vi "GetCrossSpectrumPhase.vi"(6 "calc cache":variant, 8 "error in (no error)":errorcluster, 10 "speed profile (positions [s])":sgl[](array[numeric]), 11 "waveform":waveform(sgl)) -> (0 "error out":errorcluster, 2 "channel name":string, 3 "cross phase [degrees]":cluster{"f0":dbl, "df":dbl, "phase":sgl[]}, 4 "calc cache out":variant)   [LabVIEW 2017]
uses:
  <vilib>/addons/InsightCM/Utilities/Analysis/Vibration/VibrationAnalysisFunctions.lvlib
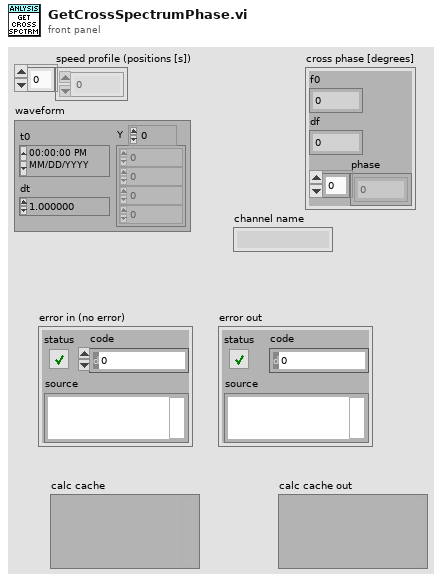
[diagram p1: front panel]
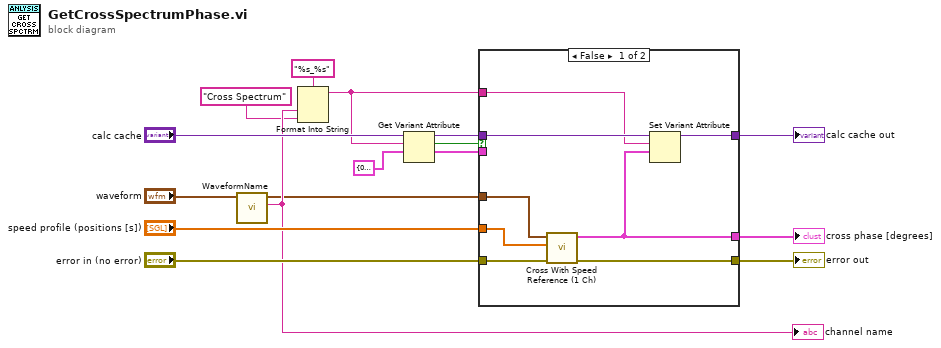
[diagram p0: block diagram]
diagram:
  n1 = call <vilib>:"WaveformName.vi"("signal in"="waveform") -> ("name"=w5:string, "signal out"=w3:waveform(sgl))  [unwired: 9 in]
  "channel name" <- w5
  n2 = Format Into String(format string="%s_%s", w5, "Cross Spectrum" ("name")) -> (resulting string=w1:string)  [unwired: 2 in, 1 out]
  n3 = Get Variant Attribute(Variant="calc cache", name=w1, default value (empty Variant)=cluster{"f0":dbl, "df":dbl, "phase":sgl[]} {"f0"=0.0, "df"=0.0, "phase"=[]} ("Cross phase [degrees]")) -> (duplicate Variant=w11:variant, found=w8:bool, value=w7:cluster{"f0":dbl, "df":dbl, "phase":sgl[]})  [unwired: 1 in, 1 out]
  n4 = case shown="False" w8 {
    tunnel: "error in (no error)" -> [w24 w27]
    tunnel: "speed profile (positions [s])" -> [w23 _]
    tunnel: [w22 w27] -> w14
    tunnel: [w18 w26] -> w13
    tunnel: w3 -> [w21 _]
    tunnel: [w19 w25] -> w10
    tunnel: w11 -> [w20 w25]
    tunnel: w1 -> [w17 _]
    tunnel: w7 -> [_ w26]
    frame False {
      n5 = call <vilib>:"Cross With Speed Reference (1 Ch).vi"("error in (no error)"=w24, "Speed Profile (Positions [s])"=w23, "Waveform"=w21) -> ("error out"=w22:errorcluster, "Cross phase [degrees]"=w18:cluster{"f0":dbl, "df":dbl, "phase":sgl[]})  [unwired: 7 in]
      n6 = Set Variant Attribute(Variant=w20, name=w17, value=w18) -> (Variant out=w19:variant)  [unwired: 1 in, 2 out]
    }
    frame True {
    }
  }
  "error out" <- w14
  "cross phase [degrees]" <- w13
  "calc cache out" <- w10
